vi "SubPanel_DataCollection_Rev11.vi"(0 "DCPowerInformationClusterArray_Input":T7(array[cluster]), 1 "VISAPowerInfoInputArray":T6(array[cluster]), 2 "Run Data SubPanel Input":T5, 3 "RF Block Parameters":T4, 4 "Oscilloscope Info Array":T3(array[cluster]) {"vertical coupling" items=["AC", "DC", "Ground"]}, 7 "error in":errorcluster) -> (20 "DCPowerInformationClusterArray_Output":T7(array[cluster]), 21 "VISAPowerInfoInputOutput":T6(array[cluster]), 22 "Run Data SubPanel Output":T5, 23 "RF Block Parameters Output":T4, 24 "Oscilloscope Info Array Output":T3(array[cluster]) {"vertical coupling" items=["AC", "DC", "Ground"]}, 27 "error out":errorcluster)   [LabVIEW 2019]
uses:
  Controls/QueueDataControl.ctl
  Controls/DataBlockControl.ctl
  Controls/RFBlockControl.ctl
  <instrlib>/niScope/Controls/niScope vertical coupling.ctl
panel:
  out "Recording Data":bool
  out "Current 2":waveform(dbl)[](graph)
  out "Voltage 2":waveform(dbl)[](graph)
  out "Current":waveform(dbl)[](graph)
  out "Voltage":waveform(dbl)[](graph)
  in  "End Collecting":bool
  out "Array":T1(array[cluster])
  in  "Begin Collecting":bool
  out "error of collection":errorcluster
  in  "exit SubVI":bool
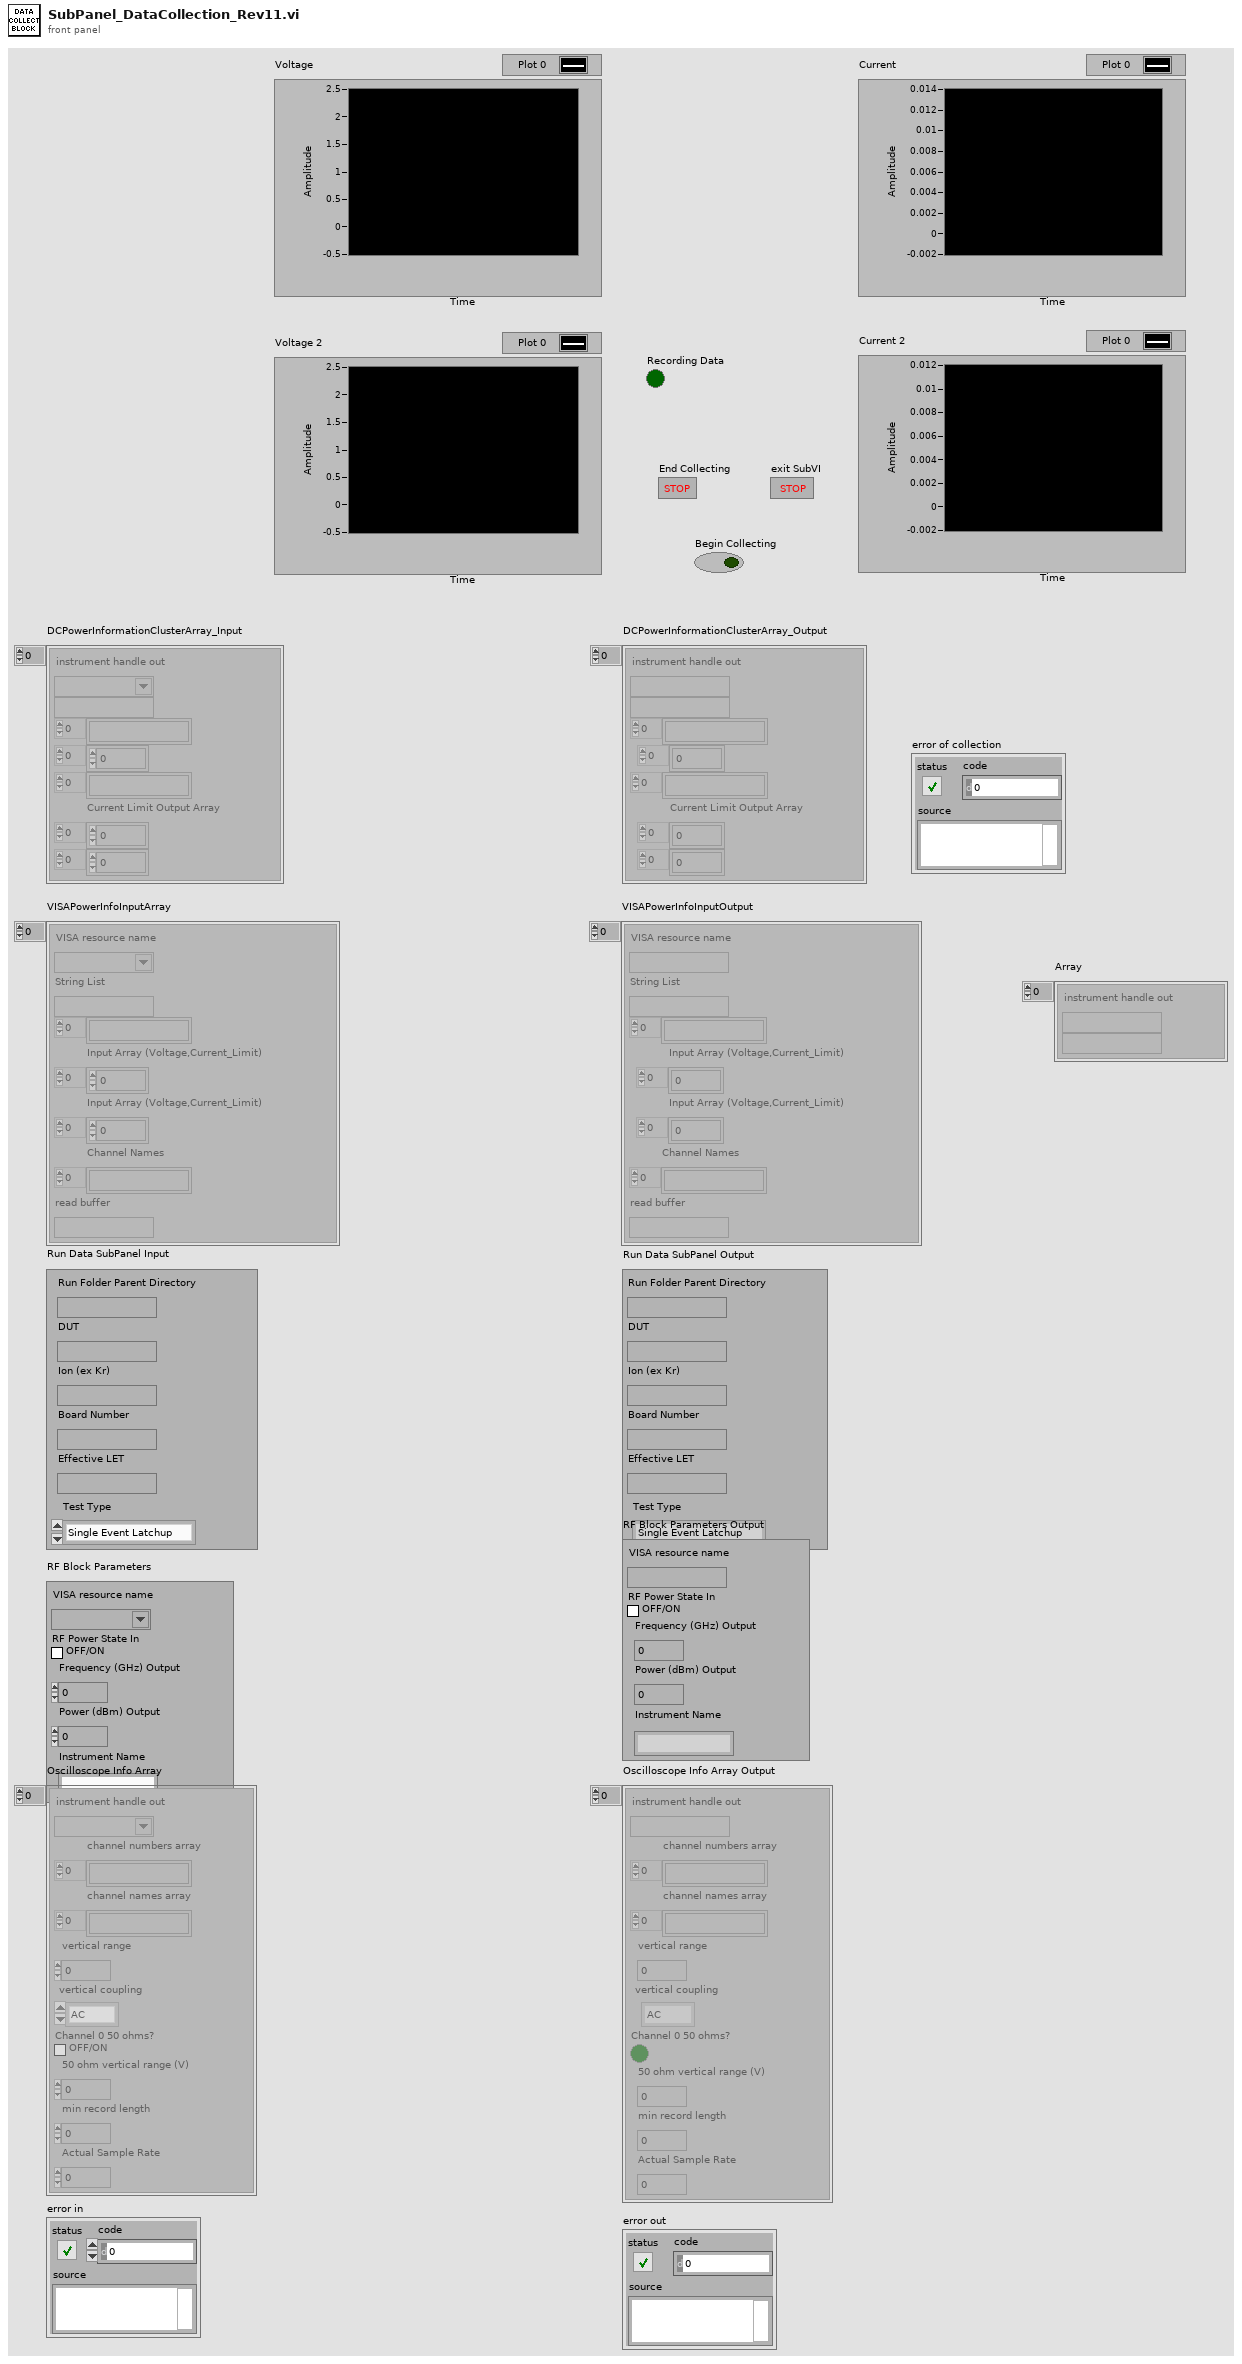
[diagram p1: front panel]
types:
  T1 = cluster{"instrument handle out":refnum<k15>, string}[]
  T2 = typedef "niScope vertical coupling.ctl" = i32
  T3 = cluster{"instrument handle out":refnum<k15>, "channel numbers array":string[], "channel names array":string[], "vertical range":dbl, "vertical coupling":T2, "Channel 0 50 ohms?":bool, "50 ohm vertical range (V)":dbl, "min record length":i32, "Actual Sample Rate":dbl}[]
  T4 = typedef "RFBlockControl.ctl" = cluster{"VISA resource name":refnum<visa-resource-name>, "RF Power State In":bool, "Frequency (GHz) Output":dbl, "Power (dBm) Output":dbl, "Instrument Name":string}
  T5 = typedef "DataBlockControl.ctl" = cluster{"Run Folder Parent Directory":path, "DUT":string, "Ion (ex Kr)":string, "Board Number":string, "Effective LET":string, "Test Type":enum16{"Single Event Latchup", "Single Event Transient", "Single Event Upset"}}
  T6 = cluster{"VISA resource name":refnum<visa-resource-name>, "String List":string, string[], "Input Array (Voltage,Current_Limit)":dbl[], "Input Array (Voltage,Current_Limit)":dbl[], "Channel Names":string[], "read buffer":string}[]
  T7 = cluster{"instrument handle out":refnum<k15>, string, string[], dbl[], string[], "Current Limit Output Array":dbl[], dbl[]}[]
  T8 = cluster{"IVI Refnum out":refnum<k15>, string, "voltage level channel 23":dbl, "Channel Name 23":string, "Current Limit":dbl, "Measure Record dt":dbl, string, "Current Threshold Reset Value Array":dbl}[]
  T9 = typedef "QueueDataControl.ctl" = cluster{"Rolling Timer":timestamp, "Initial Time":timestamp, "dt between samples":dbl[], "number of samples per fetch":i32[], "voltage measurements":dbl[][], "current measurements":dbl[][]}
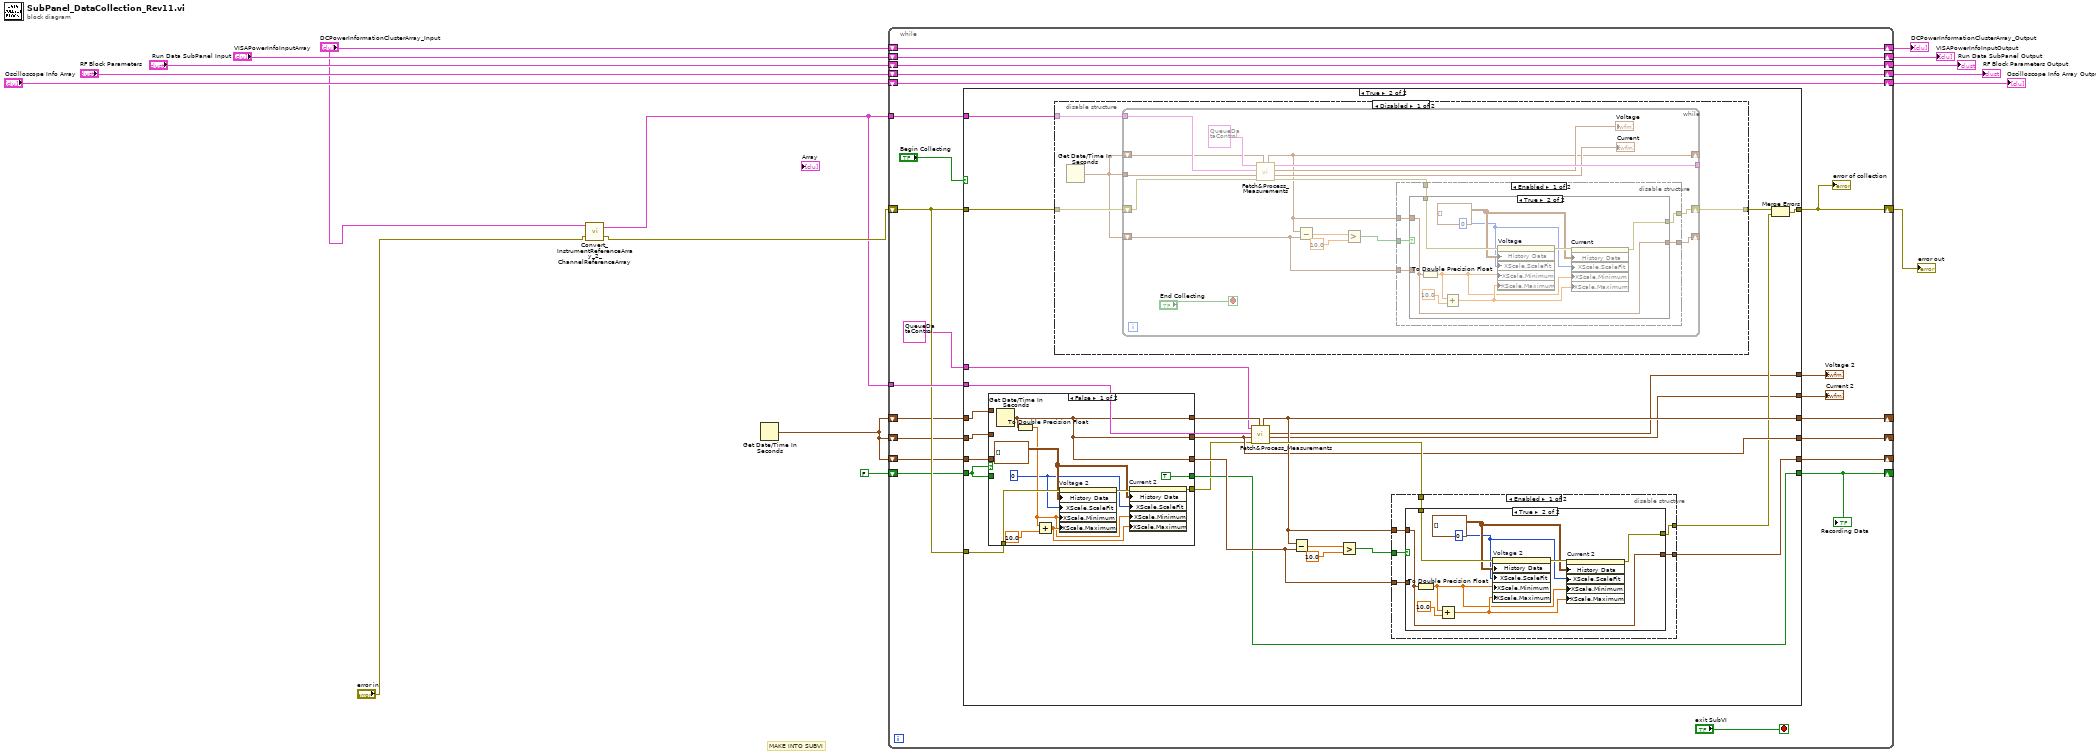
[diagram p0: block diagram]
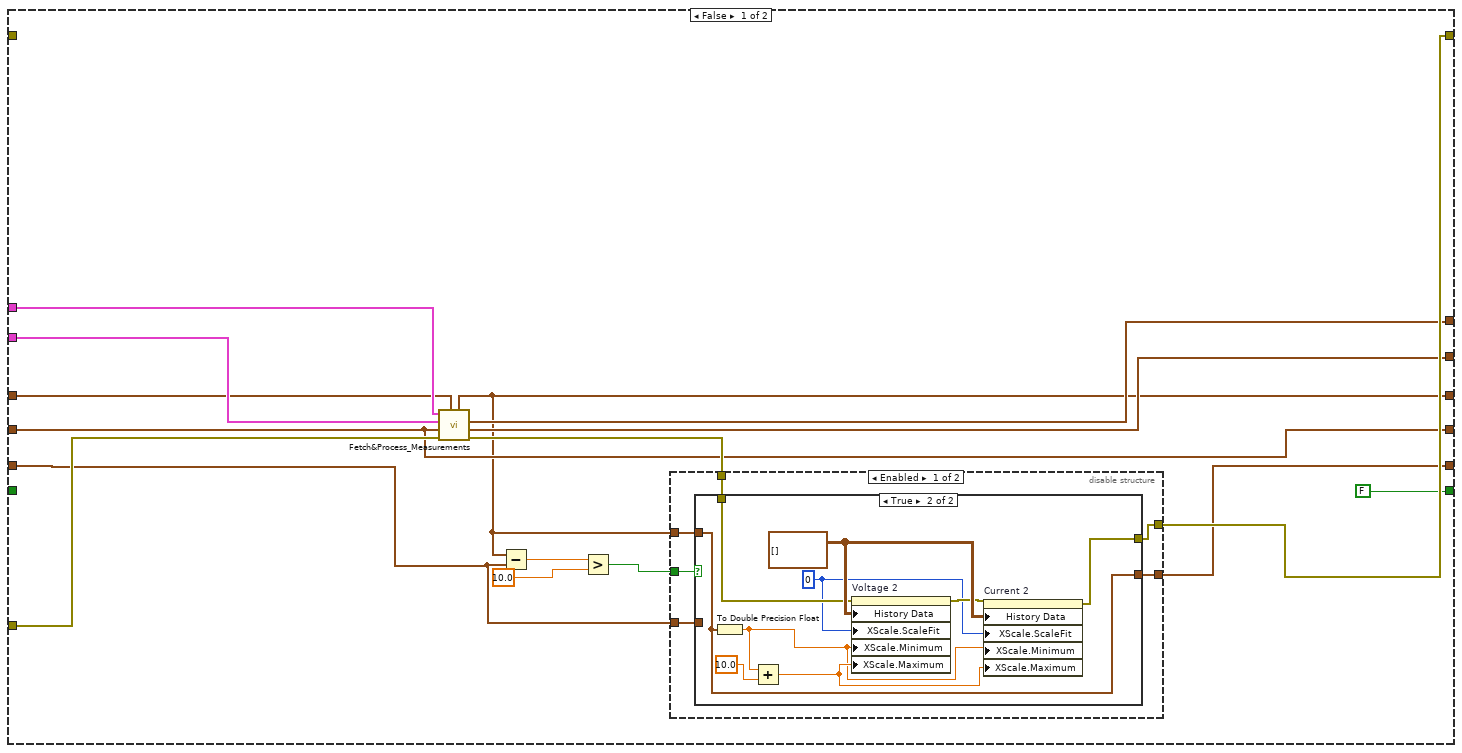
[diagram p2: hidden frame]
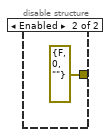
[diagram p7: hidden frame]
diagram:
  # "MAKE INTO SUBVI"
  n1 = call "Convert_InstrumentReferenceArray_2_ChannelReferenceArray.vi"("error in (no error)"="error in", "DCPowerInformationClusterArray_Input"="DCPowerInformationClusterArray_Input") -> ("error out"=w5:errorcluster, "DCPowerInformationArrayOutput"=w3:T8)
  n2 = Get Date/Time In Seconds() -> (seconds since 1Jan1904=w1:timestamp)
  n3 = while {
    shift-right: [w34] -> w16
    shift-left: "DCPowerInformationClusterArray_Input" -> [w34]
    shift-right: [w38] -> w15
    shift-left: "VISAPowerInfoInputArray" -> [w38]
    shift-right: [w37] -> w13
    shift-left: "Run Data SubPanel Input" -> [w37]
    shift-right: [w36] -> w11
    shift-left: "RF Block Parameters" -> [w36]
    shift-right: [w35] -> w9
    shift-left: "Oscilloscope Info Array" -> [w35]
    shift-right: [w33] -> w7
    shift-left: w5 -> [w28]
    tunnel: w3 -> [w30]
    tunnel: w3 -> [w29]
    shift-right: [w24] -> _
    shift-left: w1 -> [w27]
    shift-right: [w23] -> _
    shift-left: w1 -> [w26]
    shift-right: [w22] -> _
    shift-left: w1 -> [w25]
    shift-right: [w17] -> _
    shift-left: FALSE -> [w18]
    stop <- "exit SubVI" stop-if-true
    n4 = case shown="True" "Begin Collecting" {
      tunnel: w28 -> [_ w98]
      tunnel: [w46 w83] -> w33
      tunnel: w30 -> [_ w97]
      tunnel: w29 -> [w50 w92]
      tunnel: w28 -> [w47 w74]
      tunnel: w27 -> [w48 w89]
      tunnel: w26 -> [w43 w88]
      tunnel: w25 -> [w44 w87]
      tunnel: [w40 w86] -> w24
      tunnel: [w45 w85] -> w23
      tunnel: [w44 w84] -> w22
      tunnel: [w41 w80] -> w21
      tunnel: [w42 w79] -> w20
      tunnel: T9 {"Rolling Timer"=timestamp(0 s since 1904-01-01), "Initial Time"=timestamp(0 s since 1904-01-01), "dt between samples"=[], "number of samples per fetch"=[], "voltage measurements"=[], "current measurements"=[]} ("Queue Data Parameters") -> [w49 w78]
      tunnel: w18 -> [_ w76]
      tunnel: [FALSE w77] -> w17
      frame False {
        n5 = call "Fetch&Process_Measurements.vi"("Rolling Timer Input"=w48, "error in (no error)"=w47, "Initial Time"=w44, "DCPowerInformation_byChannel"=w50, "Queue Data Parameters in"=w49) -> ("error out"=w51:errorcluster, "Current Measurement"=w41:waveform(dbl)[], "Voltage Measurement"=w42:waveform(dbl)[], "Rolling Timer Output"=w40:timestamp)  [unwired: 2 in, 1 out]
        n6 = Subtract(x=w40, y=w43) -> (x-y=w53:dbl)
        n7 = Greater?(x=w53, y=10.0) -> (0:w52:bool)
        n8 = disable-structure shown="Enabled" {
          disable-tunnel: w52 -> [w60 _]
          disable-tunnel: w51 -> [w59 w73]
          disable-tunnel: [w58 w73] -> w46
          disable-tunnel: [w57 w72] -> w45
          disable-tunnel: w40 -> [w56 w72]
          disable-tunnel: w43 -> [w55 _]
          frame Enabled {
            n9 = case shown="True" w60 {
              tunnel: w59 -> [w62 w68]
              tunnel: [w62 w66] -> w58
              tunnel: [w61 w70] -> w57
              tunnel: w56 -> [_ w70]
              tunnel: w55 -> [w61 _]
              frame False {
              }
              frame True {
                w65 = u8 0 ("X Scale.Scale Fit")
                w69 = waveform(dbl)[][] [] ("History Data")
                n10 = To Double Precision Float(number=w70) -> (double precision float=w63:dbl)
                n11 = Add(x=w63, y=10.0) -> (x+y=w64:dbl)
                n12 = property on="Voltage 2" class="WFChart (strict)"(error in=w68, "History Data"=w69, "XScale.ScaleFit"=w65, "XScale.Minimum"=w63, "XScale.Maximum"=w64) -> (error out=w67:errorcluster)  [unwired: 1 in, 1 out]
                n13 = property on="Current 2" class="WFChart (strict)"(error in=w67, "History Data"=w69, "XScale.ScaleFit"=w65, "XScale.Minimum"=w63, "XScale.Maximum"=w64) -> (error out=w66:errorcluster)  [unwired: 1 in, 1 out]
              }
            }
          }
          frame Disabled {
          }
        }
      }
      frame True {
        n14 = case shown="False" w76 {
          tunnel: [w144 w153] -> w91
          tunnel: [w144 w152] -> w84
          tunnel: [w144 w154] -> w90
          tunnel: w89 -> [_ w154]
          tunnel: w88 -> [_ w153]
          tunnel: w87 -> [_ w152]
          tunnel: [TRUE w151] -> w77
          tunnel: w76 -> [_ w151]
          tunnel: [w147 w150] -> w75
          tunnel: w74 -> [w146 w150]
          frame False {
            w140 = u8 0 ("X Scale.Scale Fit")
            w145 = waveform(dbl)[][] [] ("History Data")
            n15 = Get Date/Time In Seconds() -> (seconds since 1Jan1904=w144:timestamp)
            n16 = To Double Precision Float(number=w144) -> (double precision float=w141:dbl)
            n17 = Add(x=w141, y=10.0) -> (x+y=w142:dbl)
            n18 = property on="Voltage 2" class="WFChart (strict)"(error in=w146, "History Data"=w145, "XScale.ScaleFit"=w140, "XScale.Minimum"=w141, "XScale.Maximum"=w142) -> (error out=w148:errorcluster)  [unwired: 1 in, 1 out]
            n19 = property on="Current 2" class="WFChart (strict)"(error in=w148, "History Data"=w145, "XScale.ScaleFit"=w140, "XScale.Minimum"=w141, "XScale.Maximum"=w142) -> (error out=w147:errorcluster)  [unwired: 1 in, 1 out]
          }
          frame True {
          }
        }
        n20 = disable-structure shown="Disabled" {
          disable-tunnel: w98 -> [w102 _]
          disable-tunnel: w97 -> [w101 _]
          disable-tunnel: [w100 errorcluster {"status"=FALSE, "code"=0, "source"=""} ("error out")] -> w81
          frame Disabled {
            n21 = Get Date/Time In Seconds() -> (seconds since 1Jan1904=w99:timestamp)
            n22 = while {
              shift-right: [w106] -> w100
              shift-left: w102 -> [w117]
              tunnel: w101 -> [w118]
              tunnel: w99 -> [w114]
              shift-right: [w104] -> _
              shift-left: w99 -> [w115]
              tunnel: [w113] -> _
              shift-right: [w105] -> _
              shift-left: w99 -> [w103]
              stop <- "End Collecting" stop-if-true
              n23 = call "Fetch&Process_Measurements.vi"("Rolling Timer Input"=w115, "error in (no error)"=w117, "Initial Time"=w114, "DCPowerInformation_byChannel"=w118, "Queue Data Parameters in"=T9 {"Rolling Timer"=timestamp(0 s since 1904-01-01), "Initial Time"=timestamp(0 s since 1904-01-01), "dt between samples"=[], "number of samples per fetch"=[], "voltage measurements"=[], "current measurements"=[]} ("Queue Data Parameters")) -> ("error out"=w107:errorcluster, "Current Measurement"=→"Current":waveform(dbl)[], "Voltage Measurement"=→"Voltage":waveform(dbl)[], "Queue Data Parameters out"=w113:T9, "Rolling Timer Output"=w104:timestamp)  [unwired: 2 in]
              n24 = Subtract(x=w104, y=w103) -> (x-y=w109:dbl)
              n25 = Greater?(x=w109, y=10.0) -> (0:w108:bool)
              n26 = disable-structure shown="Enabled" {
                disable-tunnel: w108 -> [w125 _]
                disable-tunnel: w107 -> [w124 w138]
                disable-tunnel: [w123 w138] -> w106
                disable-tunnel: [w122 w137] -> w105
                disable-tunnel: w104 -> [w121 w137]
                disable-tunnel: w103 -> [w120 _]
                frame Enabled {
                  n27 = case shown="True" w125 {
                    tunnel: w124 -> [w127 w136]
                    tunnel: [w127 w134] -> w123
                    tunnel: [w126 w128] -> w122
                    tunnel: w121 -> [_ w128]
                    tunnel: w120 -> [w126 _]
                    frame False {
                    }
                    frame True {
                      w131 = u8 0 ("X Scale.Scale Fit")
                      w132 = waveform(dbl)[][] [] ("History Data")
                      n28 = To Double Precision Float(number=w128) -> (double precision float=w129:dbl)
                      n29 = Add(x=w129, y=10.0) -> (x+y=w130:dbl)
                      n30 = property on="Voltage" class="WFChart (strict)"(error in=w136, "History Data"=w132, "XScale.ScaleFit"=w131, "XScale.Minimum"=w129, "XScale.Maximum"=w130) -> (error out=w135:errorcluster)  [unwired: 1 in, 1 out]
                      n31 = property on="Current" class="WFChart (strict)"(error in=w135, "History Data"=w132, "XScale.ScaleFit"=w131, "XScale.Minimum"=w129, "XScale.Maximum"=w130) -> (error out=w134:errorcluster)  [unwired: 1 in, 1 out]
                    }
                  }
                }
                frame Disabled {
                }
              }
            }
          }
          frame Enabled {
          }
        }
        n32 = call "Fetch&Process_Measurements.vi"("Rolling Timer Input"=w90, "error in (no error)"=w75, "Initial Time"=w84, "DCPowerInformation_byChannel"=w92, "Queue Data Parameters in"=w78) -> ("error out"=w93:errorcluster, "Current Measurement"=w80:waveform(dbl)[], "Voltage Measurement"=w79:waveform(dbl)[], "Rolling Timer Output"=w86:timestamp)  [unwired: 2 in, 1 out]
        n33 = Subtract(x=w86, y=w91) -> (x-y=w95:dbl)
        n34 = Greater?(x=w95, y=10.0) -> (0:w94:bool)
        n35 = disable-structure shown="Enabled" {
          disable-tunnel: w94 -> [w160 _]
          disable-tunnel: w93 -> [w159 w173]
          disable-tunnel: [w158 w173] -> w82
          disable-tunnel: [w157 w172] -> w85
          disable-tunnel: w86 -> [w156 w172]
          disable-tunnel: w91 -> [w155 _]
          frame Enabled {
            n36 = case shown="True" w160 {
              tunnel: w159 -> [w162 w171]
              tunnel: [w162 w169] -> w158
              tunnel: [w161 w163] -> w157
              tunnel: w156 -> [_ w163]
              tunnel: w155 -> [w161 _]
              frame False {
              }
              frame True {
                w166 = u8 0 ("X Scale.Scale Fit")
                w167 = waveform(dbl)[][] [] ("History Data")
                n37 = To Double Precision Float(number=w163) -> (double precision float=w164:dbl)
                n38 = Add(x=w164, y=10.0) -> (x+y=w165:dbl)
                n39 = property on="Voltage 2" class="WFChart (strict)"(error in=w171, "History Data"=w167, "XScale.ScaleFit"=w166, "XScale.Minimum"=w164, "XScale.Maximum"=w165) -> (error out=w170:errorcluster)  [unwired: 1 in, 1 out]
                n40 = property on="Current 2" class="WFChart (strict)"(error in=w170, "History Data"=w167, "XScale.ScaleFit"=w166, "XScale.Minimum"=w164, "XScale.Maximum"=w165) -> (error out=w169:errorcluster)  [unwired: 1 in, 1 out]
              }
            }
          }
          frame Disabled {
          }
        }
        n41 = Merge Errors(w81, w82) -> (w83:errorcluster)
      }
    }
    "error of collection" <- w33
    "Voltage 2" <- w20
    "Current 2" <- w21
    "Recording Data" <- w17
  }
  "DCPowerInformationClusterArray_Output" <- w16
  "VISAPowerInfoInputOutput" <- w15
  "Run Data SubPanel Output" <- w13
  "RF Block Parameters Output" <- w11
  "Oscilloscope Info Array Output" <- w9
  "error out" <- w7
